vi "一体站流程自动启动.vi"(11 "参数":T1) -> ()   [LabVIEW 2016, in "PLC.lvlib"]
uses:
  PLC.lvlib
panel:
  out "s? t:f":enum16{"初始化", "采配水启动", "仪器操作", "反冲洗", "结束"}(ring)
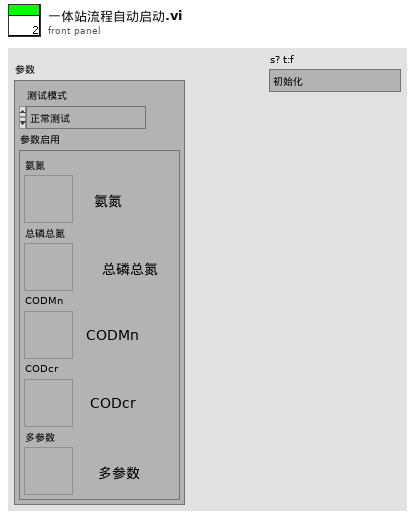
[diagram p1: front panel]
types:
  T1 = cluster{"测试模式":enum16{"正常测试", "集成干预"}, "参数启用":cluster{"氨氮":bool, "总磷总氮":bool, "CODMn":bool, "CODcr":bool, "多参数":bool}}
  T2 = cluster{"命令":string, cluster{"starting address":u16, "holding register value":u16}}
  T3 = enum16{"启动测量", "标样核查", "零点核查", "跨度核查", "空白测试", "平行样测试", "加标回收", "空白校准", "标样校准", "初始化（清洗）", "停止测试", "仪器重启", "校时", "模式设置", "测量间隔设置"}
  T4 = cluster{"时间标识":timestamp, "设备":string, "日志信息":string, "流程参数":string}
  T5 = cluster{"测量模式":enum16{"水样测量", "标样核查", "零点核查", "跨度核查", "空白测试", "加标回收", "平行样", "校零", "校标"}}
  T6 = cluster{"时间标识":timestamp, "设备":string, "日志信息":string}
  T7 = enum16{"空闲", "水样测试", "标样核查", "零点核查", "跨度核查", "空白测试", "平行样测试", "加标回收", "空白校准", "标样校准", "初始化（清洗）"}
  T8 = cluster{"R0":i16, "R1":i16, "R2":i16, "R3":i16, "R4":i16, "R5":i16, "R6":i16, "R7":i16, "R8":i16, "R9":i16, "R10":i16, "R11":i16, "R12":i16, "R13":i16, "R14":i16, "R15":i16, "R16":i16, "R17":i16, "R18":i16, "R19":i16, "R20":i16, "R21":i16, "R22":i16, "R23":i16, "R24":i16, "R25":i16, "R26":i16, "R27":i16, "R28":i16, "R29":i16, "R30":i16, "R31":i16, "R32":i16, "R33":i16, "R34":i16}
  T9 = enum32{"Bad", "Idle", "Run top level", "Running"}
  T10 = cluster{"氨氮":bool, "总磷总氮":bool, "CODMn":bool, "CODcr":bool, "多参数":bool}
  T11 = cluster{"时间标识":timestamp, "参数":string, "集成干预测试浓度值":dbl, "集成干预前测试时间":timestamp, "集成干预前测试浓度值":dbl}
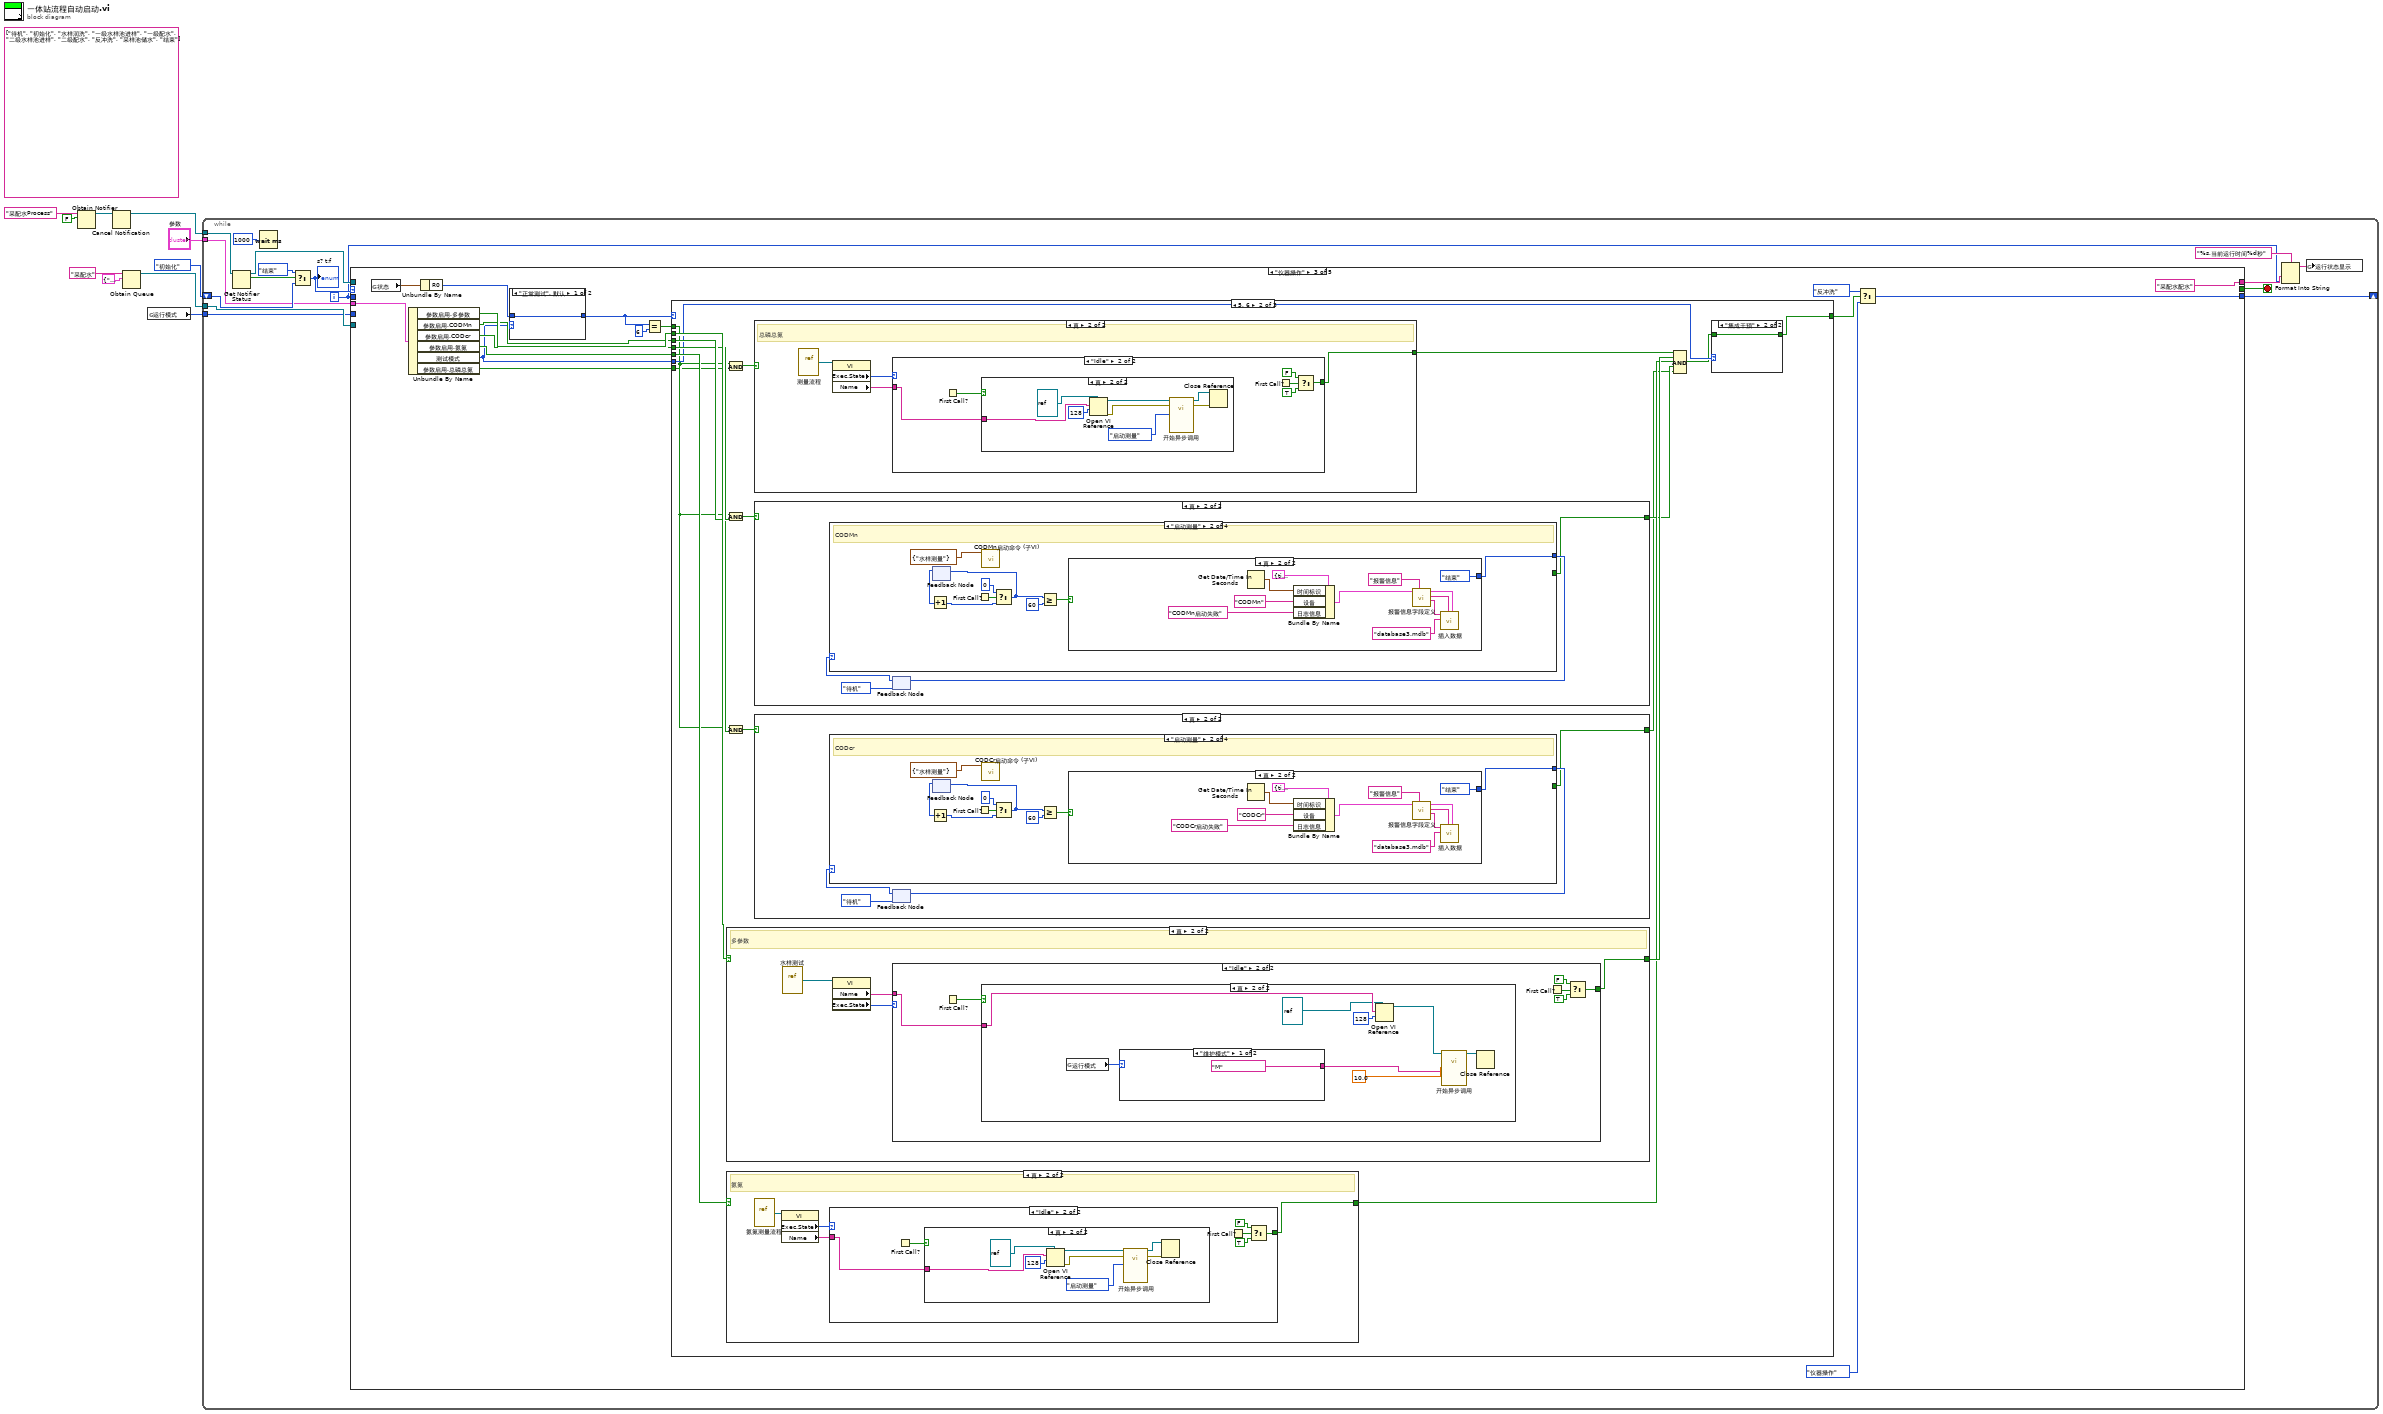
[diagram p0: block diagram]
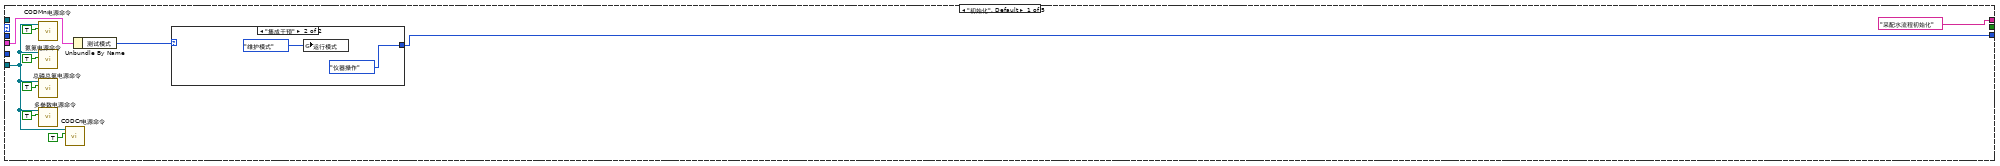
[diagram p2: hidden frame]
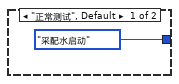
[diagram p3: hidden frame]
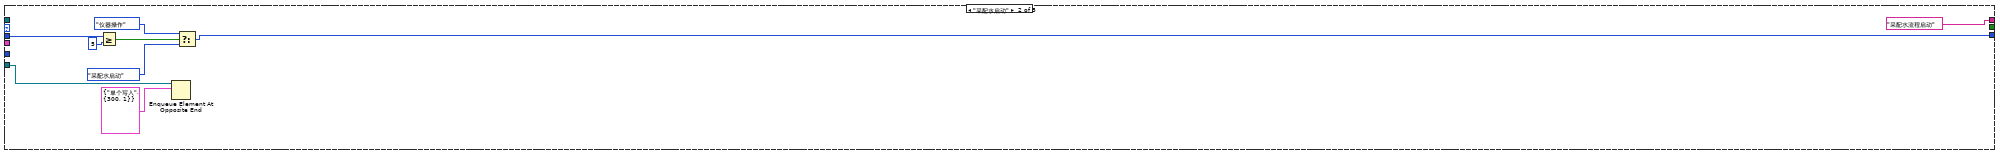
[diagram p4: hidden frame]
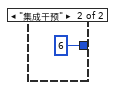
[diagram p5: hidden frame]
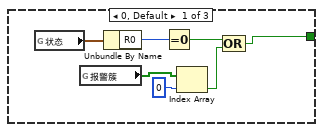
[diagram p6: hidden frame]
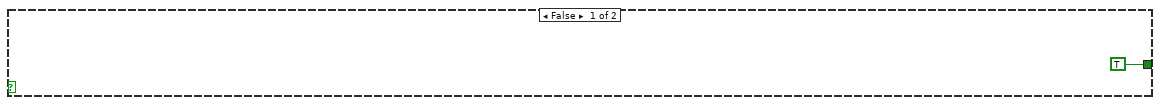
[diagram p7: hidden frame]
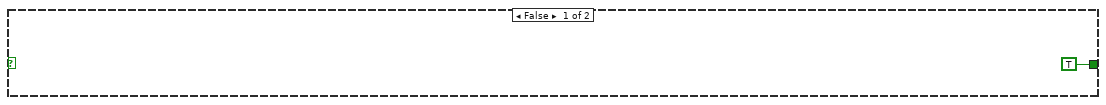
[diagram p11: hidden frame]
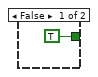
[diagram p14: hidden frame]
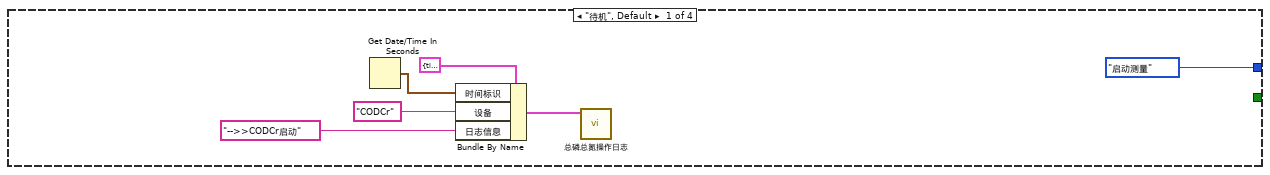
[diagram p15: hidden frame]
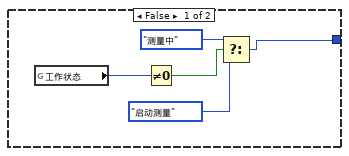
[diagram p16: hidden frame]
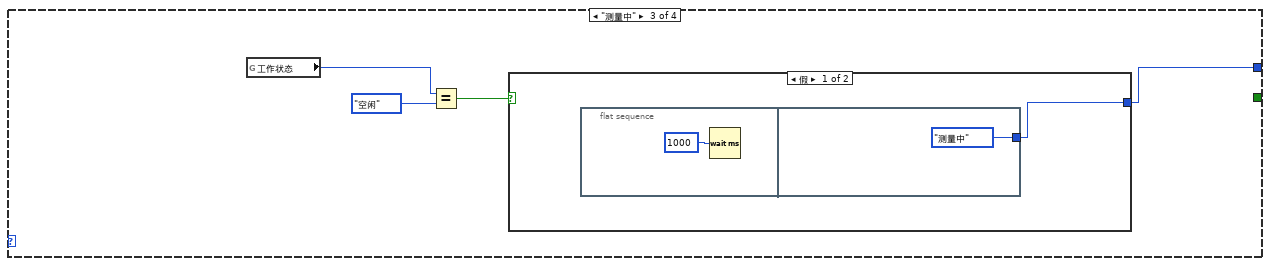
[diagram p17: hidden frame]
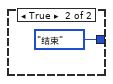
[diagram p18: hidden frame]
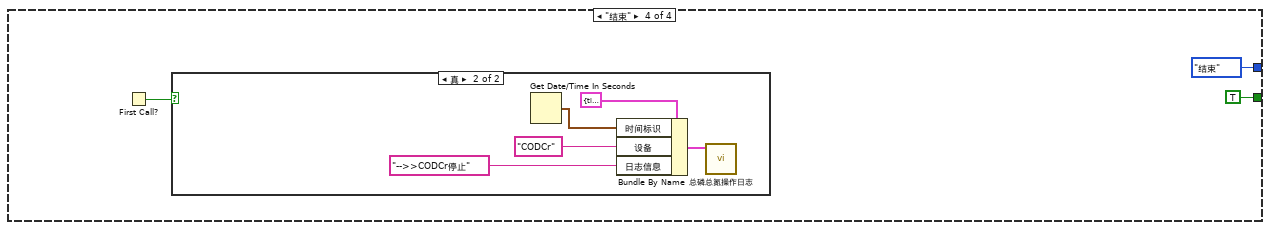
[diagram p19: hidden frame]
diagram:
  (unwired) string[][] [["待机"], ["初始化"], ["水样润洗"], ["一级水样池进样"], ["一级配水"], ["二级水样池进样"], ["二级配水"], ["反冲洗"], ["采样池储水"], ["结束"]] ("项名")
  n1 = Obtain Notifier(name (unnamed)="采配水Process" ("名称（未命名）"), notification data type=FALSE) -> (notifier out=w4:refnum<notifier>)  [unwired: 2 in, 2 out]
  n2 = Cancel Notification(0:w4) -> (8:w3:refnum<notifier>)  [unwired: 1 in, 2 out]
  n3 = Obtain Queue(name (unnamed)="采配水" ("名称（未命名）"), element data type=cluster{"命令":string, "数据":variant} {"命令"="", "数据"=variant}) -> (queue out=w7:refnum<queue>)  [unwired: 3 in, 2 out]
  n4 = global read "系统设置全局变量.vi" "运行模式"() -> (w1:enum16{"维护模式", "常规模式", "应急模式", "质控模式"})
  n5 = while {
    shift-right: [w23] -> _
    shift-left: enum16{"初始化", "采配水启动", "仪器操作", "反冲洗", "结束"}."初始化" ("枚举") -> [w19]
    tunnel: w7 -> [w26]
    tunnel: w3 -> [w22]
    tunnel: "参数" -> [w13]
    tunnel: w1 -> [w12]
    i -> [w11]
    stop <- w25 stop-if-true
    n6 = Get Notifier Status(notifier=w22) -> (notifier out=w14:refnum<notifier>, current notification=w21:bool)  [unwired: 1 in, 3 out]
    n7 = Wait (ms)(milliseconds to wait=u32 1000 ("等待时间（毫秒）")) -> ()  [unwired: 1 out]
    n8 = Select(t=enum16{"初始化", "采配水启动", "仪器操作", "反冲洗", "结束"}."结束" ("枚举"), s=w21, f=w19) -> (s? t:f=w18:enum16{"初始化", "采配水启动", "仪器操作", "反冲洗", "结束"})
    "s? t:f" <- w18
    n9 = case shown="\"仪器操作\"" w18 {
      tunnel: w26 -> [w31 w48 _ _ w419]
      tunnel: [_ _ _ _ TRUE] -> w25
      tunnel: [w30 w40 w60 w259 enum16{"初始化", "采配水启动", "仪器操作", "反冲洗", "结束"}."结束" ("枚举")] -> w23
      tunnel: ["采配水流程初始化" "采配水流程启动" "采配水配水" "等待测试完成" "采配水结束"] -> w15
      tunnel: w14 -> [_ _ _ _ w420]
      tunnel: w13 -> [w28 _ w63 w258 w416]
      tunnel: w12 -> [_ _ _ _ w415]
      tunnel: w11 -> [_ w46 _ _ _]
      frame "初始化", Default {
        n10 = call "CODMn电源命令.vi"("通电/断电"=TRUE, "队列"=w31) -> ()  [unwired: 9 in, 1 out]
        n11 = call "氨氮电源命令.vi"("通电/断电"=TRUE, "队列"=w31) -> ()  [unwired: 9 in, 1 out]
        n12 = call "总磷总氮电源命令.vi"("通电/断电"=TRUE, "队列"=w31) -> ()  [unwired: 9 in, 1 out]
        n13 = call "多参数电源命令.vi"("通电/断电"=TRUE, "队列"=w31) -> ()  [unwired: 9 in, 1 out]
        n14 = call "CODCr电源命令.vi"("通电/断电"=TRUE, "队列"=w31) -> ()  [unwired: 9 in, 1 out]
        n15 = Unbundle By Name(w28) -> ("测试模式"=w27:enum16{"正常测试", "集成干预"})
        n16 = case shown="\"集成干预\"" w27 {
          tunnel: [enum16{"初始化", "采配水启动", "仪器操作", "反冲洗", "结束"}."采配水启动" ("枚举") enum16{"初始化", "采配水启动", "仪器操作", "反冲洗", "结束"}."仪器操作" ("枚举")] -> w30
          frame "正常测试", Default {
          }
          frame "集成干预" {
            n17 = global write "系统设置全局变量.vi" "运行模式"(enum16{"维护模式", "常规模式", "应急模式", "质控模式"}."维护模式" ("运行模式")) -> ()
          }
        }
      }
      frame "采配水启动" {
        n18 = Greater Or Equal?(x=w46, y=5) -> (x >= y?=w43:bool)
        n19 = Enqueue Element At Opposite End(queue=w48, element=T2 {"命令"="单个写入", {"starting address"=300, "holding register value"=1}} ("元素")) -> ()  [unwired: 2 in, 3 out]
        n20 = Select(t=enum16{"初始化", "采配水启动", "仪器操作", "反冲洗", "结束"}."仪器操作" ("枚举"), s=w43, f=enum16{"初始化", "采配水启动", "仪器操作", "反冲洗", "结束"}."采配水启动" ("枚举")) -> (s? t:f=w40:enum16{"初始化", "采配水启动", "仪器操作", "反冲洗", "结束"})
      }
      frame "仪器操作" {
        n21 = global read "采配水全局变量.vi" "状态"() -> (w65:T8)
        n22 = Unbundle By Name(w63) -> ("参数启用.多参数"=w58:bool, "参数启用.CODMn"=w57:bool, "参数启用.CODcr"=w56:bool, "参数启用.氨氮"=w55:bool, "测试模式"=w53:enum16{"正常测试", "集成干预"}, "参数启用.总磷总氮"=w52:bool)
        n23 = Unbundle By Name(w65) -> ("R0"=w54:i16)
        n24 = case shown="\"正常测试\", 默认" w53 {
          tunnel: w54 -> [w66 _]
          tunnel: [w66 i16 6 ("R0")] -> w50
          frame "正常测试", Default {
          }
          frame "集成干预" {
          }
        }
        n25 = Equal?(x=w50, y=i16 6) -> (x = y?=w49:bool)
        n26 = case shown="5, 6" w50 {
          tunnel: [w69 w79 TRUE] -> w62
          tunnel: w58 -> [_ w91 _]
          tunnel: w57 -> [_ w90 _]
          tunnel: w56 -> [_ w87 _]
          tunnel: w55 -> [_ w86 _]
          tunnel: w49 -> [_ w78 _]
          tunnel: w53 -> [_ w81 _]
          tunnel: w52 -> [_ w77 _]
          frame 0, Default {
            n27 = global read "采配水全局变量.vi" "状态"() -> (w72:T8)
            n28 = global read "采配水全局变量.vi" "报警簇"() -> (w73:bool[])
            n29 = Unbundle By Name(w72) -> ("R0"=w71:i16)
            n30 = Equal To 0?(x=w71) -> (x = 0?=w74:bool)
            n31 = Index Array(array=w73, index=0 ("索引")) -> (element=w68:bool)
            n32 = Compound Arithmetic op=OR ("复合运算")(w74, w68) -> (w69:bool)
          }
          frame 5, 6 {
            n33 = And(x=w78, y=w77) -> (x .and. y?=w76:bool)
            n34 = And(x=w78, y=w90) -> (x .and. y?=w89:bool)
            n35 = And(x=w78, y=w87) -> (x .and. y?=w88:bool)
            n36 = case shown="真" w91 {
              tunnel: [TRUE ("t") w235] -> w85
              frame False {
              }
              frame True {
                # "多参数"
                n37 = vi-ref "水样测试.vi"() -> (w237:refnum<vi>)
                n38 = property class="VI"(reference=w237) -> ("Name"=w236:string, "Exec.State"=w238:T9)  [unwired: 1 in, 2 out]
                n39 = case shown="\"Idle\"" w238 {
                  tunnel: w236 -> [_ w244]
                  tunnel: [_ w239] -> w235
                  frame "Bad", Default {
                  }
                  frame "Idle" {
                    n40 = First Call?() -> (First Call?: T/F=w243:bool)
                    n41 = case shown="真" w243 {
                      tunnel: w244 -> [_ w251]
                      frame False {
                      }
                      frame True {
                        n42 = global read "系统设置全局变量.vi" "运行模式"() -> (w248:enum16{"维护模式", "常规模式", "应急模式", "质控模式"})
                        n43 = case shown="\"维护模式\"" w248 {
                          tunnel: ["M" ("数据标记表") "N" ("数据标记表")] -> w245
                          frame "维护模式" {
                          }
                          frame "常规模式", Default {
                          }
                        }
                        n44 = Open VI Reference(type specifier VI Refnum (for type only)=refnum<vi> refnum, vi path=w251, options=128 ("选项")) -> (vi reference=w250:refnum<vi>)  [unwired: 3 in, 1 out]
                        n45 = call-by-ref "开始异步调用"(reference=w250, "数据标记表"=w245, "水样测试时间"=10.0 ("测量时间")) -> (reference out=w249:refnum<vi>)  [unwired: 11 in, 1 out]
                        n46 = Close Reference(reference=w249) -> ()  [unwired: 1 in, 1 out]
                      }
                    }
                    n47 = First Call?() -> (First Call?: T/F=w242:bool)
                    n48 = Select(t=FALSE, s=w242, f=TRUE) -> (s? t:f=w239:bool)
                  }
                }
              }
            }
            n49 = case "条件结构" shown="真" w86 {
              tunnel: [TRUE ("t") w113] -> w84
              frame False {
              }
              frame True {
                # "氨氮"
                n50 = vi-ref "氨氮测量流程.vi"() -> (w116:refnum<vi>)
                n51 = property class="VI"(reference=w116) -> ("Exec.State"=w115:T9, "Name"=w114:string)  [unwired: 1 in, 2 out]
                n52 = case shown="\"Idle\"" w115 {
                  tunnel: w114 -> [_ w122]
                  tunnel: [_ w117] -> w113
                  frame "Bad", Default {
                  }
                  frame "Idle" {
                    n53 = First Call?() -> (First Call?: T/F=w121:bool)
                    n54 = case shown="真" w121 {
                      tunnel: w122 -> [_ w127]
                      frame False {
                      }
                      frame True {
                        n55 = Open VI Reference(type specifier VI Refnum (for type only)=refnum<vi> refnum, vi path=w127, options=128 ("选项")) -> (vi reference=w125:refnum<vi>, error out=w128:errorcluster)  [unwired: 3 in]
                        n56 = call-by-ref "开始异步调用"(reference=w125, error in=w128, "控制命令"=T3."启动测量") -> (reference out=w129:refnum<vi>, error out=w130:errorcluster)  [unwired: 11 in]
                        n57 = Close Reference(reference=w129, error in (no error)=w130) -> ()  [unwired: 1 out]
                      }
                    }
                    n58 = First Call?() -> (First Call?: T/F=w120:bool)
                    n59 = Select(t=FALSE, s=w120, f=TRUE) -> (s? t:f=w117:bool)
                  }
                }
              }
            }
            n60 = case "条件结构" shown="真" w76 {
              tunnel: [TRUE ("t") w93] -> w75
              frame False {
              }
              frame True {
                # "总磷总氮"
                n61 = vi-ref "测量流程.vi"() -> (w96:refnum<vi>)
                n62 = property class="VI"(reference=w96) -> ("Exec.State"=w95:T9, "Name"=w94:string)  [unwired: 1 in, 2 out]
                n63 = case shown="\"Idle\"" w95 {
                  tunnel: w94 -> [_ w102]
                  tunnel: [_ w97] -> w93
                  frame "Bad", Default {
                  }
                  frame "Idle" {
                    n64 = First Call?() -> (First Call?: T/F=w101:bool)
                    n65 = case shown="真" w101 {
                      tunnel: w102 -> [_ w107]
                      frame False {
                      }
                      frame True {
                        n66 = Open VI Reference(type specifier VI Refnum (for type only)=refnum<vi> refnum, vi path=w107, options=128 ("选项")) -> (vi reference=w105:refnum<vi>, error out=w108:errorcluster)  [unwired: 3 in]
                        n67 = call-by-ref "开始异步调用"(reference=w105, error in=w108, "控制命令"=T3."启动测量") -> (reference out=w109:refnum<vi>, error out=w110:errorcluster)  [unwired: 11 in]
                        n68 = Close Reference(reference=w109, error in (no error)=w110) -> ()  [unwired: 1 out]
                      }
                    }
                    n69 = First Call?() -> (First Call?: T/F=w100:bool)
                    n70 = Select(t=FALSE, s=w100, f=TRUE) -> (s? t:f=w97:bool)
                  }
                }
              }
            }
            n71 = case shown="真" w89 {
              tunnel: [TRUE w184] -> w83
              frame False {
              }
              frame True {
                n72 = feedback #1(enum16{"待机", "启动测量", "测量中", "结束"}."待机") -> (w186:enum16{"待机", "启动测量", "测量中", "结束"})
                n73 = case shown="\"启动测量\"" w186 {
                  tunnel: [enum16{"待机", "启动测量", "测量中", "结束"}."启动测量" w202 w221 enum16{"待机", "启动测量", "测量中", "结束"}."结束"] -> w185
                  tunnel: [_ _ _ TRUE] -> w184
                  frame "待机", Default {
                    n74 = Get Date/Time In Seconds() -> (seconds since 1Jan1904=w192:timestamp)
                    n75 = Bundle By Name(cluster=T4 {"时间标识"=timestamp(0 s since 1904-01-01), "设备"="", "日志信息"="", "流程参数"=""} ("data in"), "时间标识"=w192, "设备"="CODMn", "日志信息"="-->>CODMn启动") -> (w188:T4)
                    n76 = call "总磷总氮操作日志.vi"("data in"=w188) -> ()  [unwired: 11 in]
                  }
                  frame "启动测量" {
                    # "CODMn"
                    n77 = feedback #2() -> (w198:i32)  [unwired: 1 in]
                    n78 = Increment(x=w198) -> (x+1=w199:i32)
                    n79 = First Call?() -> (First Call?: T/F=w197:bool)
                    n80 = call "CODMn启动命令 (子VI).vi"("启动测量模式"=T5 {"测量模式"=enum."水样测量"}) -> ()  [unwired: 11 in]
                    n81 = Select(t=0, s=w197, f=w199) -> (s? t:f=w200:i32)
                    n82 = feedback-in #2(w200) -> ()
                    n83 = Greater Or Equal?(x=w200, y=60) -> (x >= y?=w195:bool)
                    n84 = case shown="真" w195 {
                      tunnel: [w204 enum16{"待机", "启动测量", "测量中", "结束"}."结束"] -> w202
                      frame False {
                        n85 = global read "运行时序全局变量.vi" "多列列表框"() -> (w203:i32)
                        n86 = Not Equal To 0?(x=w203) -> (x != 0?=w205:bool)
                        n87 = Select(t=enum16{"待机", "启动测量", "测量中", "结束"}."测量中", s=w205, f=enum16{"待机", "启动测量", "测量中", "结束"}."启动测量") -> (s? t:f=w204:enum16{"待机", "启动测量", "测量中", "结束"})
                      }
                      frame True {
                        n88 = Get Date/Time In Seconds() -> (seconds since 1Jan1904=w214:timestamp)
                        n89 = Bundle By Name(cluster=T6 {"时间标识"=timestamp(0 s since 1904-01-01), "设备"="", "日志信息"=""} ("data in"), "时间标识"=w214, "设备"="CODMn", "日志信息"="CODMn启动失败") -> (w208:T6)
                        n90 = call "报警信息字段定义.vi"("table输入"="报警信息", "data in"=w208) -> ("table输出"=w211:string, "columns"=w212:string[], "data out"=w213:T6)  [unwired: 7 in]
                        n91 = call "插入数据.vi"("data"=w213, "columns"=w212, "database"="database3.mdb", "table"=w211) -> ()  [unwired: 7 in, 1 out]
                      }
                    }
                  }
                  frame "测量中" {
                    n92 = global read "运行时序全局变量.vi" "多列列表框"() -> (w220:i32)
                    n93 = Equal To 0?(x=w220) -> (x = 0?=w219:bool)
                    n94 = case shown="假" w219 {
                      tunnel: [w222 enum16{"待机", "启动测量", "测量中", "结束"}."结束"] -> w221
                      frame False {
                        n95 = flat-sequence {
                          tunnel: [enum16{"待机", "启动测量", "测量中", "结束"}."测量中"] -> w222
                          frame #0 {
                            n96 = Wait (ms)(milliseconds to wait=u32 1000 ("等待时间（毫秒）")) -> ()  [unwired: 1 out]
                          }
                          frame #1 {
                          }
                        }
                      }
                      frame True {
                      }
                    }
                  }
                  frame "结束" {
                    n97 = First Call?() -> (First Call?: T/F=w226:bool)
                    n98 = case shown="真" w226 {
                      frame False {
                      }
                      frame True {
                        n99 = Get Date/Time In Seconds() -> (seconds since 1Jan1904=w233:timestamp)
                        n100 = Bundle By Name(cluster=T4 {"时间标识"=timestamp(0 s since 1904-01-01), "设备"="", "日志信息"="", "流程参数"=""} ("data in"), "时间标识"=w233, "设备"="CODMn", "日志信息"="-->>CODMn停止") -> (w229:T4)
                        n101 = call "总磷总氮操作日志.vi"("data in"=w229) -> ()  [unwired: 11 in]
                      }
                    }
                  }
                }
                n102 = feedback-in #1(w185) -> ()
              }
            }
            n103 = case shown="真" w88 {
              tunnel: [TRUE w132] -> w82
              frame False {
              }
              frame True {
                n104 = feedback #3(enum16{"待机", "启动测量", "测量中", "结束"}."待机") -> (w134:enum16{"待机", "启动测量", "测量中", "结束"})
                n105 = case shown="\"启动测量\"" w134 {
                  tunnel: [enum16{"待机", "启动测量", "测量中", "结束"}."启动测量" w150 w170 enum16{"待机", "启动测量", "测量中", "结束"}."结束"] -> w133
                  tunnel: [_ _ _ TRUE] -> w132
                  frame "待机", Default {
                    n106 = Get Date/Time In Seconds() -> (seconds since 1Jan1904=w140:timestamp)
                    n107 = Bundle By Name(cluster=T4 {"时间标识"=timestamp(0 s since 1904-01-01), "设备"="", "日志信息"="", "流程参数"=""} ("data in"), "时间标识"=w140, "设备"="CODCr", "日志信息"="-->>CODCr启动") -> (w136:T4)
                    n108 = call "总磷总氮操作日志.vi"("data in"=w136) -> ()  [unwired: 11 in]
                  }
                  frame "启动测量" {
                    # "CODcr"
                    n109 = feedback #4() -> (w146:i32)  [unwired: 1 in]
                    n110 = Increment(x=w146) -> (x+1=w147:i32)
                    n111 = First Call?() -> (First Call?: T/F=w145:bool)
                    n112 = call "CODCr启动命令 (子VI).vi"("启动测量模式"=T5 {"测量模式"=enum."水样测量"}) -> ()  [unwired: 11 in]
                    n113 = Select(t=0, s=w145, f=w147) -> (s? t:f=w148:i32)
                    n114 = feedback-in #4(w148) -> ()
                    n115 = Greater Or Equal?(x=w148, y=60) -> (x >= y?=w143:bool)
                    n116 = case shown="真" w143 {
                      tunnel: [w151 enum16{"待机", "启动测量", "测量中", "结束"}."结束"] -> w150
                      frame False {
                        n117 = global read "CODcr全局变量.vi" "工作状态"() -> (w152:T7)
                        n118 = Not Equal To 0?(x=w152) -> (x != 0?=w153:bool)
                        n119 = Select(t=enum16{"待机", "启动测量", "测量中", "结束"}."测量中", s=w153, f=enum16{"待机", "启动测量", "测量中", "结束"}."启动测量") -> (s? t:f=w151:enum16{"待机", "启动测量", "测量中", "结束"})
                      }
                      frame True {
                        n120 = Get Date/Time In Seconds() -> (seconds since 1Jan1904=w162:timestamp)
                        n121 = Bundle By Name(cluster=T6 {"时间标识"=timestamp(0 s since 1904-01-01), "设备"="", "日志信息"=""} ("data in"), "时间标识"=w162, "设备"="CODCr", "日志信息"="CODCr启动失败") -> (w156:T6)
                        n122 = call "报警信息字段定义.vi"("table输入"="报警信息", "data in"=w156) -> ("table输出"=w159:string, "columns"=w160:string[], "data out"=w161:T6)  [unwired: 7 in]
                        n123 = call "插入数据.vi"("data"=w161, "columns"=w160, "database"="database3.mdb", "table"=w159) -> ()  [unwired: 7 in, 1 out]
                      }
                    }
                  }
                  frame "测量中" {
                    n124 = global read "CODcr全局变量.vi" "工作状态"() -> (w169:T7)
                    n125 = Equal?(x=w169, y=T7."空闲" ("工作状态")) -> (x = y?=w168:bool)
                    n126 = case shown="假" w168 {
                      tunnel: [w171 enum16{"待机", "启动测量", "测量中", "结束"}."结束"] -> w170
                      frame False {
                        n127 = flat-sequence {
                          tunnel: [enum16{"待机", "启动测量", "测量中", "结束"}."测量中"] -> w171
                          frame #0 {
                            n128 = Wait (ms)(milliseconds to wait=u32 1000 ("等待时间（毫秒）")) -> ()  [unwired: 1 out]
                          }
                          frame #1 {
                          }
                        }
                      }
                      frame True {
                      }
                    }
                  }
                  frame "结束" {
                    n129 = First Call?() -> (First Call?: T/F=w175:bool)
                    n130 = case shown="真" w175 {
                      frame False {
                      }
                      frame True {
                        n131 = Get Date/Time In Seconds() -> (seconds since 1Jan1904=w182:timestamp)
                        n132 = Bundle By Name(cluster=T4 {"时间标识"=timestamp(0 s since 1904-01-01), "设备"="", "日志信息"="", "流程参数"=""} ("data in"), "时间标识"=w182, "设备"="CODCr", "日志信息"="-->>CODCr停止") -> (w178:T4)
                        n133 = call "总磷总氮操作日志.vi"("data in"=w178) -> ()  [unwired: 11 in]
                      }
                    }
                  }
                }
                n134 = feedback-in #3(w133) -> ()
              }
            }
            n135 = Compound Arithmetic op=AND ("复合运算")(w75, w85, w84, w83, w82) -> (w80:bool)
            n136 = case shown="\"集成干预\"" w81 {
              tunnel: w80 -> [_ w111]
              tunnel: [_ w111] -> w79
              frame "正常测试", Default {
              }
              frame "集成干预" {
              }
            }
          }
          frame 7..9 {
          }
        }
        n137 = Select(t=enum16{"初始化", "采配水启动", "仪器操作", "反冲洗", "结束"}."反冲洗" ("枚举"), s=w62, f=enum16{"初始化", "采配水启动", "仪器操作", "反冲洗", "结束"}."仪器操作" ("枚举")) -> (s? t:f=w60:enum16{"初始化", "采配水启动", "仪器操作", "反冲洗", "结束"})
      }
      frame "反冲洗" {
        n138 = First Call?() -> (First Call?: T/F=w256:bool)
        n139 = case shown="真" w256 {
          tunnel: w258 -> [_ w267]
          frame False {
          }
          frame True {
            n140 = Unbundle By Name(w267) -> ("测试模式"=w266:enum16{"正常测试", "集成干预"}, "参数启用"=w265:T10)
            n141 = case shown="\"集成干预\"" w266 {
              tunnel: w265 -> [w270 w354]
              frame "正常测试", Default {
                n142 = global read "系统设置全局变量.vi" "运行模式"() -> (w268:enum16{"维护模式", "常规模式", "应急模式", "质控模式"})
                n143 = global read "采配水全局变量.vi" "报警簇"() -> (w275:bool[])
                n144 = case shown="\"维护模式\"" w268 {
                  tunnel: ["M" ("table") "N" ("table")] -> w269
                  frame "维护模式" {
                  }
                  frame "常规模式", Default {
                  }
                }
                n145 = Index Array(array=w275, index #1=0 ("索引"), index #2=11 ("索引")) -> (element #1=w272:bool, element #2=w271:bool)
                n146 = case shown="真" w272 {
                  tunnel: w271 -> [w281 _]
                  tunnel: w270 -> [w280 w294]
                  tunnel: w269 -> [w278 w288]
                  frame False {
                    n147 = Unbundle By Name(w280) -> ("氨氮"=w279:bool)
                    n148 = case shown="真" w281 {
                      tunnel: w279 -> [_ w283]
                      tunnel: w278 -> [_ w282]
                      frame False {
                      }
                      frame True {
                        n149 = case shown="真" w283 {
                          tunnel: w282 -> [_ w284]
                          tunnel: [_ w285] -> _
                          frame False {
                          }
                          frame True {
                            n150 = call "取水点无水样数据存储.vi"("数据标识"="lw", "数据类型"=w284, "table"="氨氮") -> ("error out"=w285:errorcluster)  [unwired: 8 in]
                          }
                        }
                      }
                    }
                  }
                  frame True {
                    n151 = Unbundle By Name(w294) -> ("氨氮"=w293:bool, "CODMn"=w292:bool, "CODcr"=w291:bool, "多参数"=w290:bool, "总磷总氮"=w289:bool)
                    n152 = case shown="真" w293 {
                      tunnel: w288 -> [_ w346]
                      tunnel: [_ w347] -> _
                      frame False {
                      }
                      frame True {
                        n153 = call "取水点无水样数据存储.vi"("数据标识"="Z", "数据类型"=w346, "table"="氨氮") -> ("error out"=w347:errorcluster)  [unwired: 8 in]
                      }
                    }
                    n154 = case shown="真" w292 {
                      tunnel: w288 -> [_ w343]
                      tunnel: [_ w342] -> _
                      frame False {
                      }
                      frame True {
                        n155 = call "取水点无水样数据存储.vi"("数据标识"="Z", "数据类型"=w343, "table"="CODMn") -> ("error out"=w342:errorcluster)  [unwired: 8 in]
                      }
                    }
                    n156 = case shown="真" w291 {
                      tunnel: w288 -> [_ w339]
                      tunnel: [_ w338] -> _
                      frame False {
                      }
                      frame True {
                        n157 = call "取水点无水样数据存储.vi"("数据标识"="Z", "数据类型"=w339, "table"="CODCr") -> ("error out"=w338:errorcluster)  [unwired: 8 in]
                      }
                    }
                    n158 = case shown="真" w289 {
                      tunnel: w288 -> [_ w296]
                      tunnel: [_ w295] -> _
                      frame False {
                      }
                      frame True {
                        n159 = call "取水点无水样数据存储.vi"("数据标识"="Z", "数据类型"=w296, "table"="总氮") -> ("error out"=w297:errorcluster)  [unwired: 8 in]
                        n160 = call "取水点无水样数据存储.vi"("error in (no error)"=w297, "数据标识"="Z", "数据类型"=w296, "table"="总磷") -> ("error out"=w295:errorcluster)  [unwired: 7 in]
                      }
                    }
                    n161 = case shown="真" w290 {
                      tunnel: w288 -> [_ w309]
                      frame False {
                      }
                      frame True {
                        n162 = global read "断电保存变量.vi" "Cond"() -> (w304:bool)
                        n163 = global read "断电保存变量.vi" "Turb"() -> (w305:bool)
                        n164 = global read "断电保存变量.vi" "DO"() -> (w306:bool)
                        n165 = global read "断电保存变量.vi" "pH"() -> (w307:bool)
                        n166 = global read "断电保存变量.vi" "藻密度"() -> (w302:bool)
                        n167 = global read "断电保存变量.vi" "Temp"() -> (w308:bool)
                        n168 = case shown="真" w307 {
                          tunnel: w309 -> [_ w331]
                          tunnel: [_ w330] -> _
                          frame False {
                          }
                          frame True {
                            n169 = call "取水点无水样数据存储.vi"("数据标识"="Z", "数据类型"=w331, "table"="pH") -> ("error out"=w330:errorcluster)  [unwired: 8 in]
                          }
                        }
                        n170 = case shown="真" w306 {
                          tunnel: w309 -> [_ w327]
                          tunnel: [_ w326] -> _
                          frame False {
                          }
                          frame True {
                            n171 = call "取水点无水样数据存储.vi"("数据标识"="Z", "数据类型"=w327, "table"="DO") -> ("error out"=w326:errorcluster)  [unwired: 8 in]
                          }
                        }
                        n172 = case shown="真" w305 {
                          tunnel: w309 -> [_ w319]
                          tunnel: [_ w318] -> _
                          frame False {
                          }
                          frame True {
                            n173 = call "取水点无水样数据存储.vi"("数据标识"="Z", "数据类型"=w319, "table"="浊度") -> ("error out"=w318:errorcluster)  [unwired: 8 in]
                          }
                        }
                        n174 = case shown="真" w304 {
                          tunnel: w309 -> [_ w323]
                          tunnel: [_ w322] -> _
                          frame False {
                          }
                          frame True {
                            n175 = call "取水点无水样数据存储.vi"("数据标识"="Z", "数据类型"=w323, "table"="比电导率") -> ("error out"=w322:errorcluster)  [unwired: 8 in]
                          }
                        }
                        n176 = global read "断电保存变量.vi" "叶绿素a启用"() -> (w303:bool)
                        n177 = case shown="真" w308 {
                          tunnel: w309 -> [_ w335]
                          tunnel: [_ w334] -> _
                          frame False {
                          }
                          frame True {
                            n178 = call "取水点无水样数据存储.vi"("数据标识"="Z", "数据类型"=w335, "table"="水温") -> ("error out"=w334:errorcluster)  [unwired: 8 in]
                          }
                        }
                        n179 = case shown="真" w302 {
                          tunnel: w309 -> [_ w311]
                          tunnel: [_ w310] -> _
                          frame False {
                          }
                          frame True {
                            n180 = call "取水点无水样数据存储.vi"("数据标识"="Z", "数据类型"=w311, "table"="藻密度") -> ("error out"=w310:errorcluster)  [unwired: 8 in]
                          }
                        }
                        n181 = case shown="真" w303 {
                          tunnel: w309 -> [_ w315]
                          tunnel: [_ w314] -> _
                          frame False {
                          }
                          frame True {
                            n182 = call "取水点无水样数据存储.vi"("数据标识"="Z", "数据类型"=w315, "table"="叶绿素") -> ("error out"=w314:errorcluster)  [unwired: 8 in]
                          }
                        }
                      }
                    }
                  }
                }
              }
              frame "集成干预" {
                n183 = Unbundle By Name(w354) -> ("氨氮"=w353:bool, "CODMn"=w352:bool, "CODcr"=w351:bool, "多参数"=w350:bool)
                n184 = case shown="真" w353 {
                  frame False {
                  }
                  frame True {
                    n185 = call "获取最近两组水样测试数据.vi"("table"="氨氮") -> ("error out"=w412:errorcluster, "存储变量"=w413:T11)  [unwired: 9 in]
                    n186 = call "集成干预测试数据存储.vi"("error in (no error)"=w412, "存储变量"=w413) -> ("error out"=w408:errorcluster)  [unwired: 9 in]
                    n187 = call "获取最近两组水样测试数据.vi"("error in (no error)"=w408, "table"="总磷") -> ("error out"=w411:errorcluster, "存储变量"=w410:T11)  [unwired: 8 in]
                    n188 = call "集成干预测试数据存储.vi"("error in (no error)"=w411, "存储变量"=w410) -> ()  [unwired: 9 in, 1 out]
                  }
                }
                n189 = case shown="真" w352 {
                  frame False {
                  }
                  frame True {
                    n190 = call "获取最近两组水样测试数据.vi"("table"="CODMn") -> ("error out"=w405:errorcluster, "存储变量"=w406:T11)  [unwired: 9 in]
                    n191 = call "集成干预测试数据存储.vi"("error in (no error)"=w405, "存储变量"=w406) -> ()  [unwired: 9 in, 1 out]
                  }
                }
                n192 = case shown="真" w351 {
                  frame False {
                  }
                  frame True {
                    n193 = call "获取最近两组水样测试数据.vi"("table"="CODCr") -> ("error out"=w402:errorcluster, "存储变量"=w403:T11)  [unwired: 9 in]
                    n194 = call "集成干预测试数据存储.vi"("error in (no error)"=w402, "存储变量"=w403) -> ()  [unwired: 9 in, 1 out]
                  }
                }
                n195 = case shown="真" w350 {
                  frame False {
                  }
                  frame True {
                    n196 = global read "断电保存变量.vi" "Temp"() -> (w361:bool)
                    n197 = case shown="真" w361 {
                      tunnel: [_ w398] -> w367
                      frame False {
                      }
                      frame True {
                        n198 = call "获取最近两组水样测试数据.vi"("table"="水温") -> ("error out"=w401:errorcluster, "存储变量"=w400:T11)  [unwired: 9 in]
                        n199 = call "集成干预测试数据存储.vi"("error in (no error)"=w401, "存储变量"=w400) -> ("error out"=w398:errorcluster)  [unwired: 9 in]
                      }
                    }
                    n200 = global read "断电保存变量.vi" "pH"() -> (w360:bool)
                    n201 = case shown="真" w360 {
                      tunnel: [_ w394] -> w366
                      tunnel: w367 -> [_ w393]
                      frame False {
                      }
                      frame True {
                        n202 = call "获取最近两组水样测试数据.vi"("error in (no error)"=w393, "table"="pH") -> ("error out"=w397:errorcluster, "存储变量"=w396:T11)  [unwired: 8 in]
                        n203 = call "集成干预测试数据存储.vi"("error in (no error)"=w397, "存储变量"=w396) -> ("error out"=w394:errorcluster)  [unwired: 9 in]
                      }
                    }
                    n204 = global read "断电保存变量.vi" "DO"() -> (w359:bool)
                    n205 = case shown="真" w359 {
                      tunnel: [_ w389] -> w365
                      tunnel: w366 -> [_ w388]
                      frame False {
                      }
                      frame True {
                        n206 = call "获取最近两组水样测试数据.vi"("error in (no error)"=w388, "table"="DO") -> ("error out"=w392:errorcluster, "存储变量"=w391:T11)  [unwired: 8 in]
                        n207 = call "集成干预测试数据存储.vi"("error in (no error)"=w392, "存储变量"=w391) -> ("error out"=w389:errorcluster)  [unwired: 9 in]
                      }
                    }
                    n208 = global read "断电保存变量.vi" "Cond"() -> (w358:bool)
                    n209 = case shown="真" w358 {
                      tunnel: [_ w384] -> w364
                      tunnel: w365 -> [_ w383]
                      frame False {
                      }
                      frame True {
                        n210 = call "获取最近两组水样测试数据.vi"("error in (no error)"=w383, "table"="比电导率") -> ("error out"=w387:errorcluster, "存储变量"=w386:T11)  [unwired: 8 in]
                        n211 = call "集成干预测试数据存储.vi"("error in (no error)"=w387, "存储变量"=w386) -> ("error out"=w384:errorcluster)  [unwired: 9 in]
                      }
                    }
                    n212 = global read "断电保存变量.vi" "Turb"() -> (w357:bool)
                    n213 = case shown="真" w357 {
                      tunnel: [_ w379] -> w363
                      tunnel: w364 -> [_ w378]
                      frame False {
                      }
                      frame True {
                        n214 = call "获取最近两组水样测试数据.vi"("error in (no error)"=w378, "table"="浊度") -> ("error out"=w382:errorcluster, "存储变量"=w381:T11)  [unwired: 8 in]
                        n215 = call "集成干预测试数据存储.vi"("error in (no error)"=w382, "存储变量"=w381) -> ("error out"=w379:errorcluster)  [unwired: 9 in]
                      }
                    }
                    n216 = global read "断电保存变量.vi" "叶绿素a启用"() -> (w356:bool)
                    n217 = case shown="真" w356 {
                      tunnel: [_ w374] -> w362
                      tunnel: w363 -> [_ w373]
                      frame False {
                      }
                      frame True {
                        n218 = call "获取最近两组水样测试数据.vi"("error in (no error)"=w373, "table"="叶绿素") -> ("error out"=w377:errorcluster, "存储变量"=w376:T11)  [unwired: 8 in]
                        n219 = call "集成干预测试数据存储.vi"("error in (no error)"=w377, "存储变量"=w376) -> ("error out"=w374:errorcluster)  [unwired: 9 in]
                      }
                    }
                    n220 = global read "断电保存变量.vi" "藻密度"() -> (w355:bool)
                    n221 = case shown="真" w355 {
                      tunnel: [_ w369] -> _
                      tunnel: w362 -> [_ w368]
                      frame False {
                      }
                      frame True {
                        n222 = call "获取最近两组水样测试数据.vi"("error in (no error)"=w368, "table"="藻密度") -> ("error out"=w372:errorcluster, "存储变量"=w371:T11)  [unwired: 8 in]
                        n223 = call "集成干预测试数据存储.vi"("error in (no error)"=w372, "存储变量"=w371) -> ("error out"=w369:errorcluster)  [unwired: 9 in]
                      }
                    }
                  }
                }
              }
            }
          }
        }
        n224 = global read "采配水全局变量.vi" "状态"() -> (w264:T8)
        n225 = Unbundle By Name(w264) -> ("R0"=w263:i16)
        n226 = Equal To 0?(x=w263) -> (x = 0?=w262:bool)
        n227 = Select(t=enum16{"初始化", "采配水启动", "仪器操作", "反冲洗", "结束"}."结束" ("枚举"), s=w262, f=enum16{"初始化", "采配水启动", "仪器操作", "反冲洗", "结束"}."反冲洗" ("枚举")) -> (s? t:f=w259:enum16{"初始化", "采配水启动", "仪器操作", "反冲洗", "结束"})
      }
      frame "结束" {
        n228 = Release Queue(queue=w419) -> ()  [unwired: 2 in, 3 out]
        n229 = Unbundle By Name(w416) -> ("测试模式"=w417:enum16{"正常测试", "集成干预"})
        n230 = Cancel Notification(0:w420) -> (8:w421:refnum<notifier>)  [unwired: 1 in, 2 out]
        n231 = Release Notifier(notifier=w421) -> ()  [unwired: 2 in, 3 out]
        n232 = case shown="\"集成干预\"" w417 {
          tunnel: w415 -> [_ w424]
          frame "正常测试", Default {
          }
          frame "集成干预" {
            n233 = global write "系统设置全局变量.vi" "运行模式"(w424) -> ()
          }
        }
      }
    }
    n234 = Format Into String(format string="%s,当前运行时间%d秒" ("格式字符串"), w15, w11) -> (resulting string=w16:string)  [unwired: 2 in, 1 out]
    n235 = global write "采配水全局变量.vi" "运行状态显示"(w16) -> ()
  }
